vi "Strain Page.vi"(8 "error in (no error)":errorcluster, 11 "Node Ptr":T4 format="%.0x") -> (0 "error out":errorcluster)   [LabVIEW 2010, in "PXIe-433x Custom Device.lvlib"]
uses:
  PXIe-433x Custom Device.lvlib
  Strain Bridge Information.ctl
  Strain Information.ctl
  <vilib>/NI Veristand/Custom Device API/Custom Device Item Ref.ctl
  Max Value.ctl
  Min Value.ctl
  Board Info for checking settings.ctl
  Sensor Type.ctl
  Global.vi
  <vilib>/NI VeriStand/Custom Device API/Get Item Property (Variant).vi
  <vilib>/NI VeriStand/Custom Device API/Get Item Property (Double).vi
  <vilib>/NI Veristand/Custom Device API/Set Item Property (Variant).vi
  <vilib>/NI Veristand/Custom Device API/Set Item Property (Double).vi
  <vilib>/NI Veristand/Custom Device API/Custom Device API.lvlib
panel:
  in  "Board Info for checking":T1
  in  "Minimum Value":T2=-0.05 caption="Strain"
  in  "Maximum Value":T3=0.05 caption="Strain"
  out "Error Description":string
  out "Tab Control":enum32{"No Error", "No Check", "Error"}(tab)
  out "Valid":bool=TRUE
  in  "No Error Check Details":bool
  out "No Check":bool=TRUE
  in  "Error Details":bool
  out "Valid Configuration?":bool
  in  "stop":bool
  in  "strain gage information":T5={"gage factor"=2.0, "nominal gage resistance"=350.0, "poisson ratio"=0.3} {"nominal gage resistance" format="%0.2f"; "poisson ratio" format="%0.2f"; "gage factor" format="%0.2f"}
  in  "bridge information":T6={"strain configuration"=10183, "lead wire resistance"=0.0, "initial bridge voltage"=0.0, "voltage excitation source"=10200, "voltage excitation value"=2.5} {"initial bridge voltage" format="%0.2f"; "voltage excitation source" items=["Internal"=10200, "External"=10167, "None"=10230]; "voltage excitation value" format="%0.2f"; "lead wire resistance" format="%0.2f"; "strain configuration" items=["Full Bridge I"=10183, "Full Bridge II"=10184, "Full Bridge III"=10185, "Half Bridge I"=10188, "Half Bridge II"=10189, "Quarter Bridge I"=10271, "Quarter Bridge II"=10272]}
  # "No Error"
  # "No Error"
  # "No Error Check"
  # "No Error Check"
  # "Error!"
  # "Error!"
  # "Ohm"
  # "V"
  # "V"
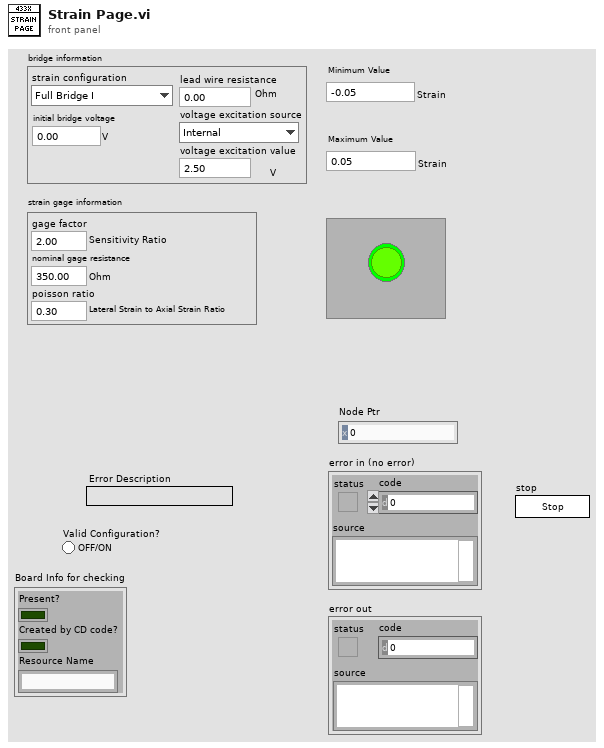
[diagram p1: front panel]
types:
  T1 = typedef "PXIe-433x Custom Device.lvlib/Board Info for checking settings.ctl" = cluster{"Present?":bool, "Created by CD code?":bool, "Resource Name":string}
  T2 = typedef "PXIe-433x Custom Device.lvlib/Min Value.ctl" = dbl
  T3 = typedef "PXIe-433x Custom Device.lvlib/Max Value.ctl" = dbl
  T4 = typedef "Custom Device API.lvlib/Custom Device Item Ref.ctl" = u64
  T5 = typedef "PXIe-433x Custom Device.lvlib/Strain Information.ctl" = cluster{"gage factor":dbl, "nominal gage resistance":dbl, "poisson ratio":dbl}
  T6 = typedef "PXIe-433x Custom Device.lvlib/Strain Bridge Information.ctl" = cluster{"strain configuration":i32, "lead wire resistance":dbl, "initial bridge voltage":dbl, "voltage excitation source":i32, "voltage excitation value":dbl}
  T7 = typedef "PXIe-433x Custom Device.lvlib/Sensor Type.ctl" = enum16{"Strain", "Force", "Pressure", "Torque"}
  T8 = typedef "Custom Device API.lvlib/Custom Device Commands.ctl" = enum16{"Default", "Item renamed", "Shutdown", "Dynamic button pressed"}
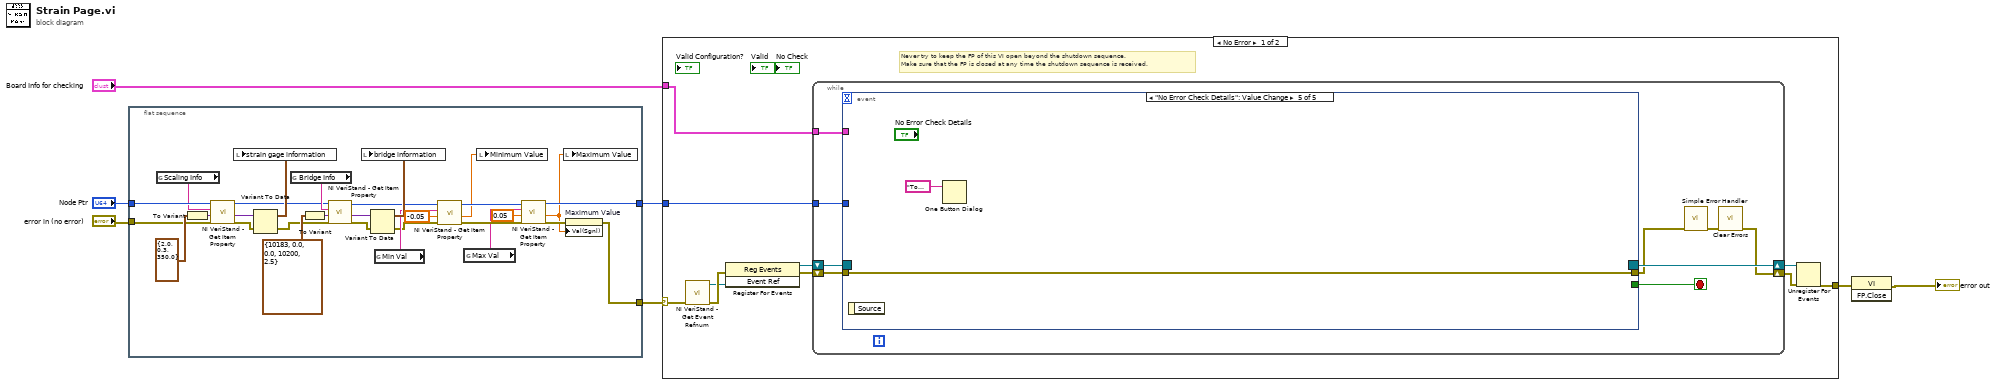
[diagram p0: block diagram]
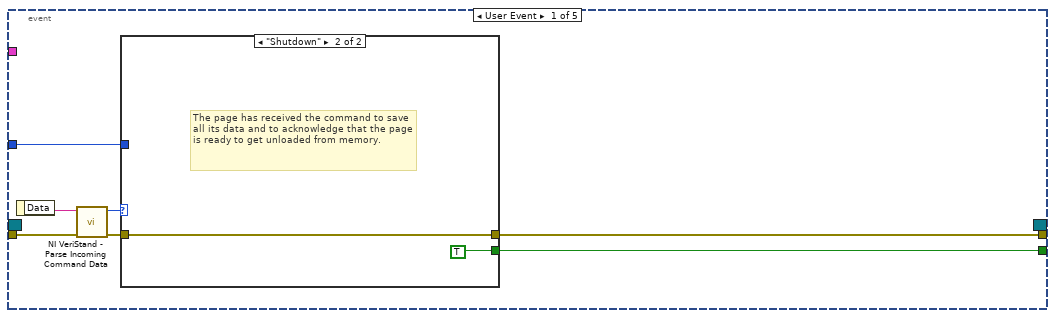
[diagram p2: hidden frame]
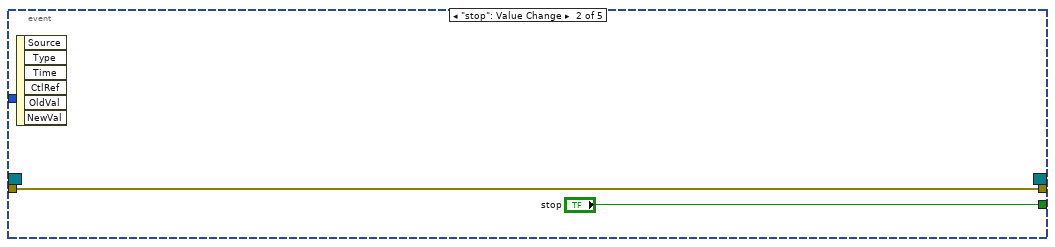
[diagram p4: hidden frame]
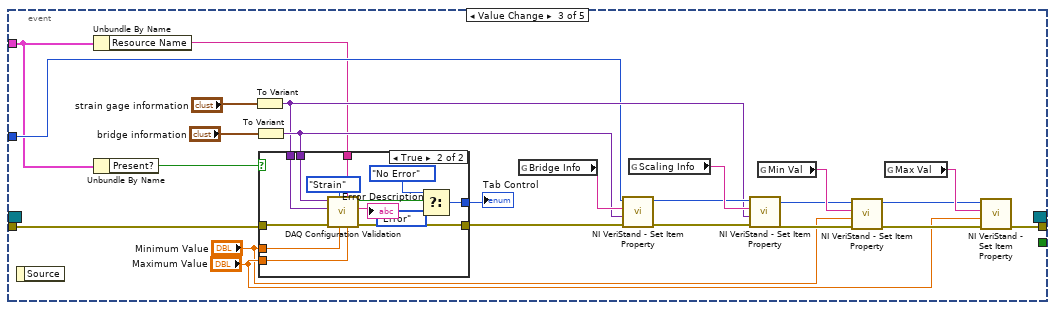
[diagram p5: hidden frame]
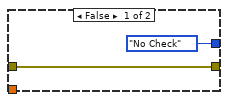
[diagram p6: hidden frame]
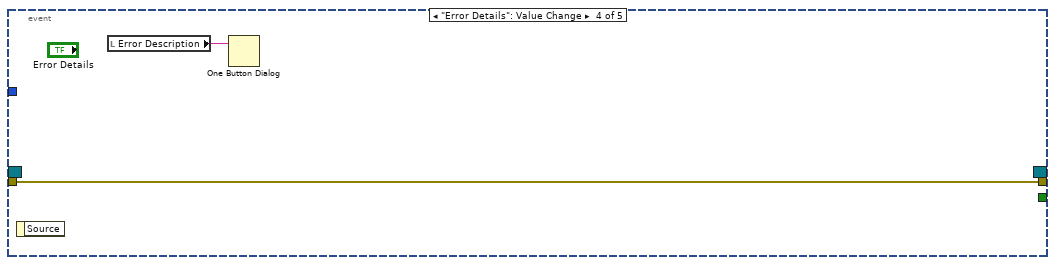
[diagram p7: hidden frame]
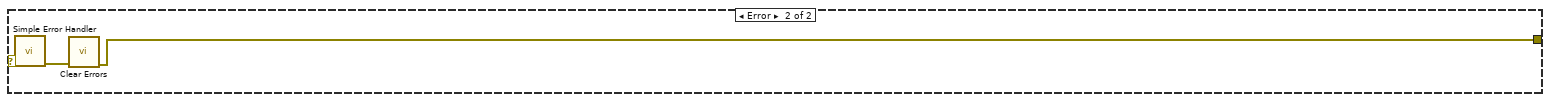
[diagram p8: hidden frame]
diagram:
  n1 = flat-sequence {
    tunnel: [w18] -> w5
    tunnel: "Node Ptr" -> [w36]
    tunnel: [w10] -> w2
    tunnel: "error in (no error)" -> [w8]
    frame #0 {
      n2 = global read "Global.vi" "Scaling Info"() -> (w35:string)
      n3 = To Variant(anything=T5 {"gage factor"=2.0, "nominal gage resistance"=0.3, "poisson ratio"=350.0} ("strain gage information")) -> (Variant=w33:variant)
      n4 = call-poly <vilib>:"NI VeriStand - Get Item Property.vi"("error in (no error)"=w8, "Default Value"=w33, "Property Name"=w35, "Item Ref in"=w36) -> ("error out"=w14:errorcluster, "Value"=w32:variant, "Item Ref out"=w28:T4)  [unwired: 4 in, 1 out]
      n5 = Variant To Data(error in=w14, Variant=w32) -> (error out=w13:errorcluster, data=w31:T5)  [unwired: 1 in]
      n6 = local write "strain gage information"(w31) -> ()
      n7 = global read "Global.vi" "Bridge Info"() -> (w30:string)
      n8 = To Variant(anything=T6 {"strain configuration"=10183, "lead wire resistance"=0.0, "initial bridge voltage"=0.0, "voltage excitation source"=10200, "voltage excitation value"=2.5} ("bridge information")) -> (Variant=w26:variant)
      n9 = call-poly <vilib>:"NI VeriStand - Get Item Property.vi"("error in (no error)"=w13, "Default Value"=w26, "Property Name"=w30, "Item Ref in"=w28) -> ("error out"=w12:errorcluster, "Value"=w29:variant, "Item Ref out"=w19:T4)  [unwired: 4 in, 1 out]
      n10 = Variant To Data(error in=w12, Variant=w29) -> (error out=w17:errorcluster, data=w25:T6)  [unwired: 1 in]
      n11 = local write "bridge information"(w25) -> ()
      n12 = global read "Global.vi" "Min Val"() -> (w20:string)
      n13 = call-poly <vilib>:"NI VeriStand - Get Item Property.vi"("error in (no error)"=w17, "Default Value"=-0.05, "Property Name"=w20, "Item Ref in"=w19) -> ("error out"=w23:errorcluster, "Value"=w22:dbl, "Item Ref out"=w24:T4)  [unwired: 4 in, 1 out]
      n14 = global read "Global.vi" "Max Val"() -> (w21:string)
      n15 = local write "Minimum Value"(w22) -> ()
      n16 = call-poly <vilib>:"NI VeriStand - Get Item Property.vi"("error in (no error)"=w23, "Default Value"=0.05, "Property Name"=w21, "Item Ref in"=w24) -> ("error out"=w11:errorcluster, "Value"=w9:dbl, "Item Ref out"=w18:T4)  [unwired: 4 in, 1 out]
      n17 = local write "Maximum Value"(w9) -> ()
      n18 = property on="Maximum Value" class="DigNum (strict)"(error in=w11, "Val(Sgnl)"=w9) -> (error out=w10:errorcluster)  [unwired: 1 in, 1 out]
    }
  }
  n19 = case shown="No Error" w2 {
    selector: w2 -> [w38 w113]
    tunnel: [w43 w111] -> w7
    tunnel: w5 -> [w39 _]
    tunnel: "Board Info for checking" -> [w37 _]
    frame No Error {
      # "Never try to keep the FP of this VI open beyond the shutdown sequence.\nMake sure that the FP is closed at any time the shutdown sequence is received."
      n20 = call <vilib>:"NI VeriStand - Get Event Refnum.vi"("error in (no error)"=w38) -> ("error out"=w46:errorcluster, "Event Ref"=w42:refnum<user-event>)  [unwired: 9 out]
      n21 = register-events(error in=w46, w42) -> (reference out=w40:refnum<event-registration>, error out=w41:errorcluster)  [unwired: 1 in]
      n22 = while {
        tunnel: w39 -> [w52]
        shift-right: [w49] -> w44
        shift-left: w41 -> [w54]
        shift-right: [w55] -> w45
        shift-left: w40 -> [w53]
        tunnel: w37 -> [w47]
        stop <- w48 stop-if-true
        n23 = event shown="[4] \"No Error Check Details\": Value Change" {
          selector: w53 -> [_ _ _ _ _]
          dyn-events: [_ _ _ _ _] -> w55
          timeout: _ -> [_ _ _ _ _]
          tunnel: w54 -> [w62 w66 w89 w107 w110]
          tunnel: [w58 "stop" _ _ _] -> w48
          tunnel: [w57 w66 w74 w107 w110] -> w51
          tunnel: w52 -> [w56 _ w70 _ _]
          tunnel: w47 -> [_ _ w69 _ _]
          event User Event {
            n24 = event-data() -> ("Data"=w61:string)  [unwired: 1 out]
            n25 = call <vilib>:"NI VeriStand - Parse Incoming Command Data.vi"("error in (no error)"=w62, "Data"=w61) -> ("error out"=w60:errorcluster, "Action"=w59:T8)  [unwired: 8 out]
            n26 = case shown="\"Shutdown\"" w59 {
              tunnel: w60 -> [w63 w64]
              tunnel: [_ TRUE] -> w58
              tunnel: [w63 w64] -> w57
              tunnel: w56 -> [_ _]
              frame "Default", Default {
              }
              frame "Shutdown" {
                # "The page has received the command to save all its data and to acknowledge that the page is ready to get unloaded from memory."
              }
            }
          }
          event "stop": Value Change {
            n27 = event-data() -> ()  [unwired: 7 out]
          }
          event Value Change {
            n28 = event-data() -> ()  [unwired: 2 out]
            n29 = Unbundle By Name(w69) -> ("Resource Name"=w68:string)
            n30 = Unbundle By Name(w69) -> ("Present?"=w90:bool)
            n31 = To Variant(anything="strain gage information") -> (Variant=w80:variant)
            n32 = To Variant(anything="bridge information") -> (Variant=w84:variant)
            n33 = case shown="True" w90 {
              tunnel: w89 -> [w93 w106]
              tunnel: [w93 w99] -> w85
              tunnel: "Minimum Value" -> [_ w104]
              tunnel: "Maximum Value" -> [_ w103]
              tunnel: w80 -> [_ w101]
              tunnel: w84 -> [_ w102]
              tunnel: [enum32{"No Error", "No Check", "Error"}."No Check" ("Tab Control") w97] -> w91
              tunnel: w68 -> [_ w94]
              frame False {
              }
              frame True {
                n34 = call "DAQ Configuration Validation.vi"("Maximum Value"=w103, "DAQ Resource Name"=w94, "Minimum Value"=w104, "Sensor Type"=Sensor_Type."Strain", "error in"=w106, "scaling info"=w101, "bridge info"=w102) -> ("error IO"=w99:errorcluster, "Error Source"=→"Error Description":string, "Valid configuration?"=w95:bool)  [unwired: 2 in]
                n35 = Select(t=enum32{"No Error", "No Check", "Error"}."No Error" ("Tab Control"), s=w95, f=enum32{"No Error", "No Check", "Error"}."Error" ("Tab Control")) -> (s? t:f=w97:enum32{"No Error", "No Check", "Error"})
              }
            }
            "Tab Control" <- w91
            n36 = global read "Global.vi" "Bridge Info"() -> (w86:string)
            n37 = call-poly <vilib>:"NI VeriStand - Set Item Property.vi"("error in (no error)"=w85, "Value"=w84, "Property Name"=w86, "Item Ref in"=w70) -> ("error out"=w81:errorcluster, "Item Ref out"=w82:T4)  [unwired: 5 in, 1 out]
            n38 = global read "Global.vi" "Scaling Info"() -> (w83:string)
            n39 = call-poly <vilib>:"NI VeriStand - Set Item Property.vi"("error in (no error)"=w81, "Value"=w80, "Property Name"=w83, "Item Ref in"=w82) -> ("error out"=w78:errorcluster, "Item Ref out"=w77:T4)  [unwired: 5 in, 1 out]
            n40 = global read "Global.vi" "Min Val"() -> (w79:string)
            n41 = call-poly <vilib>:"NI VeriStand - Set Item Property.vi"("error in (no error)"=w78, "Value"="Minimum Value", "Property Name"=w79, "Item Ref in"=w77) -> ("error out"=w75:errorcluster, "Item Ref out"=w73:T4)  [unwired: 5 in, 1 out]
            n42 = global read "Global.vi" "Max Val"() -> (w76:string)
            n43 = call-poly <vilib>:"NI VeriStand - Set Item Property.vi"("error in (no error)"=w75, "Value"="Maximum Value", "Property Name"=w76, "Item Ref in"=w73) -> ("error out"=w74:errorcluster)  [unwired: 5 in, 2 out]
          }
          event "Error Details": Value Change {
            n44 = event-data() -> ()  [unwired: 2 out]
            n45 = local read "Error Description"() -> (w108:string)
            n46 = One Button Dialog(message=w108) -> ()  [unwired: 1 in, 1 out]
          }
          event "No Error Check Details": Value Change {
            n47 = event-data() -> ()  [unwired: 2 out]
            n48 = One Button Dialog(message="To perform error checking during Edition time, code needs either a physical local PXIe-433x or simulated one. One simulated couldn't be created, no error checking will be performed while editing settings. Error checking will still be performed while deploying Custom-Device.") -> ()  [unwired: 1 in, 1 out]
          }
        }
        n49 = call <vilib>:"Simple Error Handler.vi"("error in (no error)"=w51) -> ("error out"=w50:errorcluster)  [unwired: 1 in, 7 out]
        n50 = call <vilib>:"Clear Errors.vi"("error in (no error)"=w50) -> ("error out"=w49:errorcluster)  [unwired: 6 out]
      }
      n51 = Unregister For Events(event registration refnum=w45, error in=w44) -> (error out=w43:errorcluster)
    }
    frame Error {
      n52 = call <vilib>:"Simple Error Handler.vi"("error in (no error)"=w113) -> ("error out"=w112:errorcluster)  [unwired: 1 in, 7 out]
      n53 = call <vilib>:"Clear Errors.vi"("error in (no error)"=w112) -> ("error out"=w111:errorcluster)  [unwired: 6 out]
    }
  }
  n54 = invoke class="VI" method="FP.Close"(error in=w7) -> (error out=→"error out":errorcluster)  [unwired: 2 in, 2 out]
